vi "Read status.vi"(8 "error in (no error)":errorcluster, 11 "_cameraBase in":refnum<class "_cameraBase.lvclass">) -> (0 "error out":errorcluster, 2 "status":bool, 3 "_cameraBase out":refnum<class "_cameraBase.lvclass">)   [LabVIEW 2018, in "_cameraBase.lvclass"]
uses:
  _cameraBase.lvclass
  _cameraBase.lvclass/_cameraBase.ctl
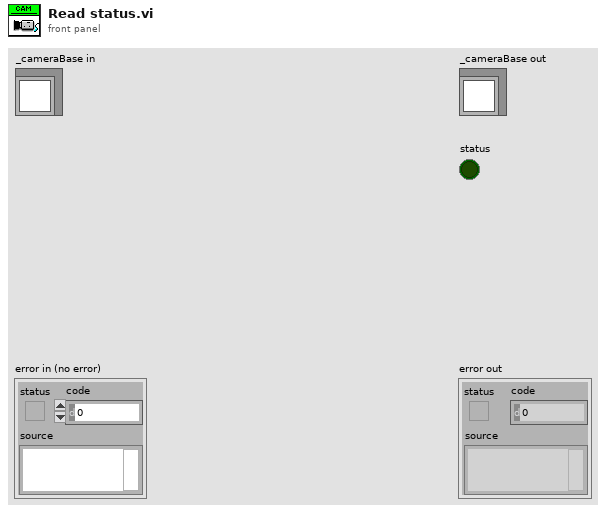
[diagram p1: front panel]
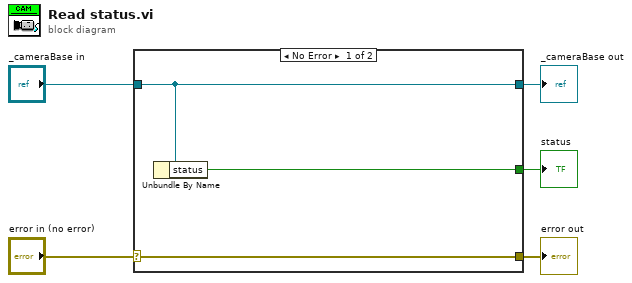
[diagram p0: block diagram]
diagram:
  n1 = case shown="No Error" "error in (no error)" {
    selector: "error in (no error)" -> [w8 w9]
    tunnel: [w8 w9] -> w4
    tunnel: [w7 w10] -> w2
    tunnel: "_cameraBase in" -> [w7 w10]
    tunnel: [w6 _] -> w1
    frame No Error {
      n2 = Unbundle By Name(w7) -> ("status"=w6:bool)
    }
    frame Error {
    }
  }
  "error out" <- w4
  "_cameraBase out" <- w2
  "status" <- w1
